vi "EdgeDetect_File.vi"(0 "Image Path":path=path "/Users/milandahal/Desktop/a.png", 5 "did":string="aa5f5cb08903b53f224287e0", 7 "wid":string="e1f73355bdbd9a727fdd999e", 9 "eid":string, 11 "Scaling Factor":dbl) -> (4 "Device Out":T2, 6 "Comm":T1, 8 "image":picture, 15 "error out":errorcluster)   [LabVIEW 2019]
uses:
  <userlib>/Onshape/_SubVI/Cluster.ctl
  <userlib>/IoT Devices/_subVIs/HTTPComm.ctl
  <userlib>/Onshape/_SubVI/z did wid and eid.vi
  <userlib>/OnshapeFeatureFunctions/Onshape Feature Funcrions/_SubVI/FS Sketch Polyline.vi
  <userlib>/OnshapeFeatureFunctions/Onshape Feature Funcrions/_SubVI/FS Operation Extrude.vi
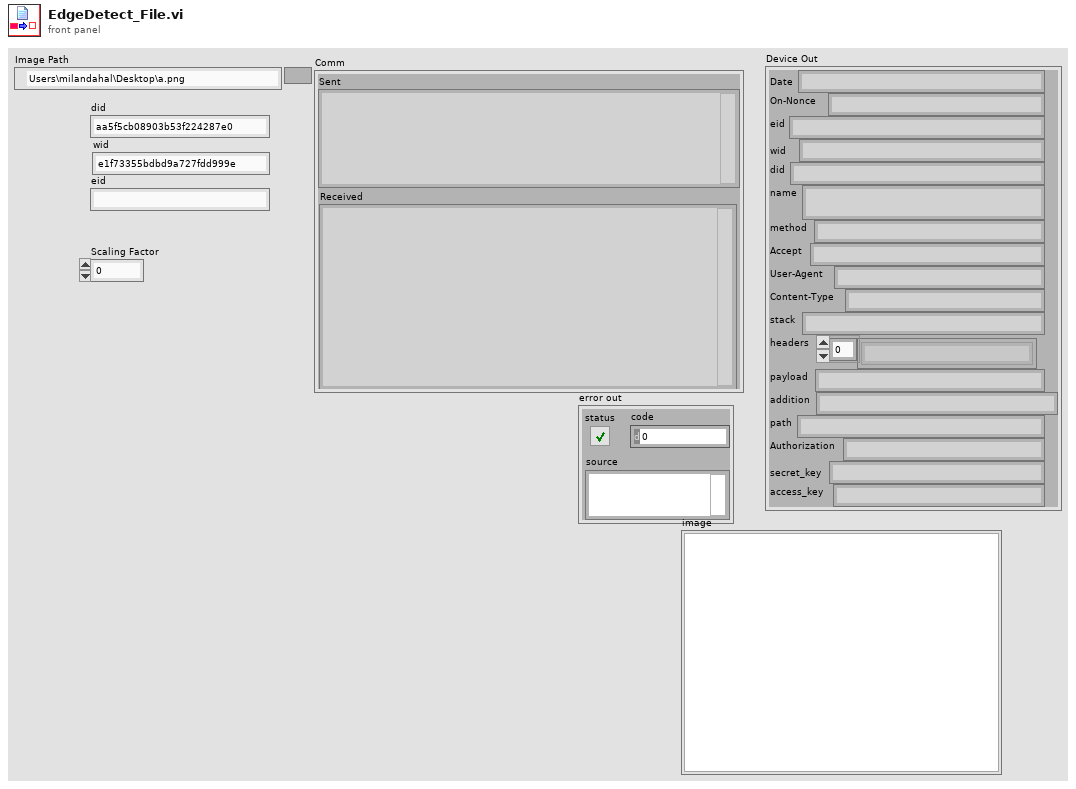
[diagram p1: front panel]
types:
  T1 = typedef "HTTPComm.ctl" = cluster{"url":string, "sent headers":string, "sent body":string, "headers":string, "body":string, "Sent":string, "Received":string}
  T2 = typedef "Cluster.ctl" = cluster{"Date":string, "On-Nonce":string, "eid":string, "wid":string, "did":string, "name":string, "method":string, "Accept":string, "User-Agent":string, "Content-Type":string, "stack":string, "headers":string[], "payload":string, "addition":string, "path":string, "Authorization":string, "secret_key":string, "access_key":string}
  T3 = typedef "QT_Image.ctl" = cluster{"Width":i32, "Height":i32, "Depth":i32, "data":u8[], "Compressed data":u8[], "Color table":u32[], "Duration":i32, "Options":i32, "Timestamp":i32, "ID":i32, "Reserved":i32, "Dialogs":u32}
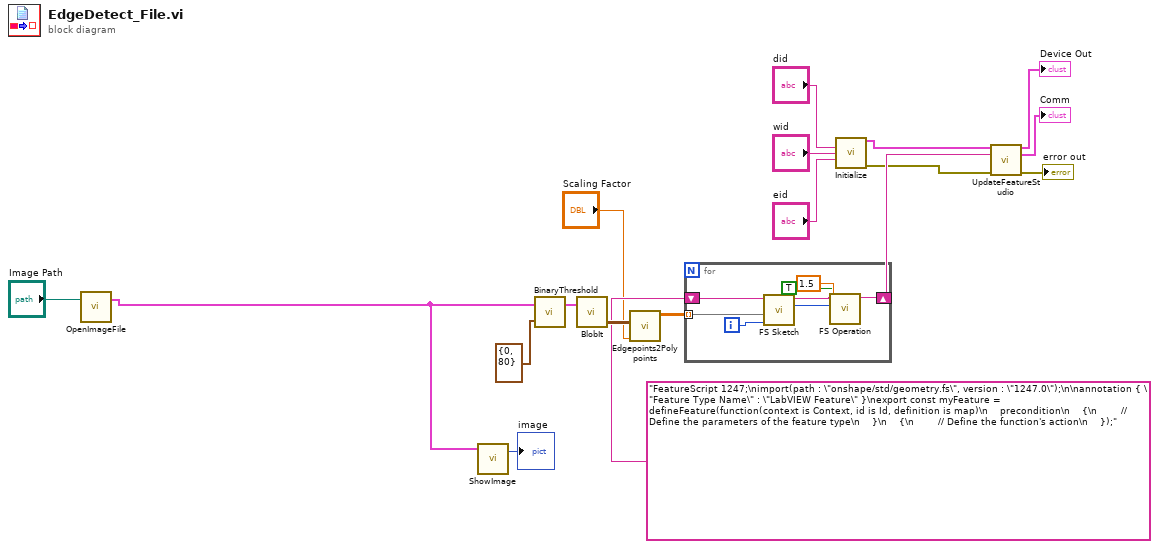
[diagram p0: block diagram]
diagram:
  n1 = call <userlib>:"OpenImageFile.vi"("selected path"="Image Path") -> ("Image Out"=w3:T3)  [unwired: 2 in]
  n2 = call <userlib>:"ShowImage.vi"("Image"=w3) -> ("image"=→"image":picture)  [unwired: 2 in, 1 out]
  n3 = call <userlib>:"BinaryThreshold.vi"("threshold"=cluster{u8, u8} {0, 80}, "Image In"=w3) -> ("Image Out"=w1:T3)  [unwired: 1 in]
  n4 = call <userlib>:"BlobIt.vi"("Image in"=w1) -> ("Array 2"=w18:cluster{"Row":i32, "Col":i32}[][])  [unwired: 1 in, 2 out]
  n5 = call <userlib>:"Edgepoints2Polypoints.vi"("Scaling Factor"="Scaling Factor", "Edgepoints In"=w18) -> ("Polyline Out"=w17:dbl[][][])  [unwired: 9 in]
  n6 = for {
    tunnel: w17 -> [w25] mode=indexing
    shift-right: [w22] -> w12
    shift-left: "FeatureScript 1247;\nimport(path : \"onshape/std/geometry.fs\", version : \"1247.0\");\n\nannotation { \"Feature Type Name\" : \"LabVIEW Feature\" }\nexport const myFeature = defineFeature(function(context is Context, id is Id, definition is map)\n    precondition\n    {\n        // Define the parameters of the feature type\n    }\n    {\n        // Define the function's action\n    });" ("Feature In") -> [w24]
    i -> [w19]
    n7 = call-poly <userlib>:"FS Sketch.vi"("Sketch #"=w19, "Polyline Points"=w25, "Feature In"=w24) -> ("Feature Out"=w23:string)  [unwired: 8 in]
    n8 = call-poly <userlib>:"FS Operation.vi"("Ignore Inner Loops?"=TRUE, "Extrude Depth"=1.5, "Sketch # to Extrude"=w19, "Feature In"=w23) -> ("Feature Out"=w22:string)  [unwired: 7 in]
  }
  n9 = call-poly <userlib>:"Initialize.vi"("did"="did", "wid"="wid", "eid"="eid") -> ("Device Out"=w13:T2, "error out"=w5:errorcluster)  [unwired: 11 in]
  n10 = call <userlib>:"UpdateFeatureStudio.vi"("Device In"=w13, "FeatureScript"=w12, "error in"=w5) -> ("Device Out"=→"Device Out":T2, "Comm"=→"Comm":T1, "error out"=→"error out":errorcluster)  [unwired: 10 in]
